vi "Dispatch_Chunks_to_Threads.vi"(4 "[IN] # rows last transfer":i32, 5 "[IN] # rows single transfer":i32, 6 "[IN] Number of threads":i32, 7 "[IN] Number of chunks":i32) -> (0 "[OUT] Remained rows last transfer":i32, 1 "[OUT] Rows of img for port":i32, 2 "[OUT] Dispatched lastly":i32, 3 "[OUT] Dispatched chunks":i32)   [LabVIEW 2020]
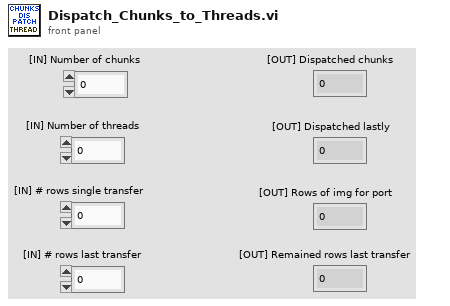
[diagram p1: front panel]
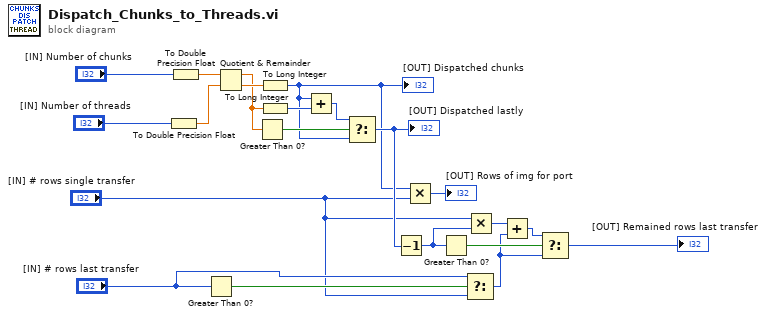
[diagram p0: block diagram]
diagram:
  n1 = To Double Precision Float(number="[IN] Number of threads") -> (double precision float=w16:dbl)
  n2 = To Double Precision Float(number="[IN] Number of chunks") -> (double precision float=w19:dbl)
  n3 = Greater Than 0?(x="[IN] # rows last transfer") -> (x > 0?=w11:bool)
  n4 = Quotient & Remainder(x=w19, y=w16) -> (x-y*floor(x/y)=w4:dbl, floor(x/y)=w18:dbl)
  n5 = Greater Than 0?(x=w4) -> (x > 0?=w17:bool)
  n6 = To Long Integer(number=w18) -> (32bit integer=w2:i32)
  "[OUT] Dispatched chunks" <- w2
  n7 = To Long Integer(number=w4) -> (32bit integer=w3:i32)
  n8 = Add(x=w2, y=w3) -> (x+y=w1:i32)
  n9 = Select(t=w1, s=w17, f=w2) -> (s? t:f=w14:i32)
  "[OUT] Dispatched lastly" <- w14
  n10 = Decrement(x=w14) -> (x-1=w12:i32)
  n11 = Multiply(x=w2, y="[IN] # rows single transfer") -> (x*y=→"[OUT] Rows of img for port":i32)
  n12 = Greater Than 0?(x=w12) -> (x > 0?=w13:bool)
  n13 = Select(t="[IN] # rows last transfer", s=w11, f="[IN] # rows single transfer") -> (s? t:f=w6:i32)
  n14 = Multiply(x="[IN] # rows single transfer", y=w12) -> (x*y=w10:i32)
  n15 = Add(x=w10, y=w6) -> (x+y=w7:i32)
  n16 = Select(t=w7, s=w13, f=w6) -> (s? t:f=→"[OUT] Remained rows last transfer":i32)
